vi "2016110576강재원_1번Project.vi"() -> ()   [LabVIEW 2017]
uses:
  <vilib>/DAQmx/read.llb/DAQmx Read (Analog DBL 1Chan 1Samp).vi
  <vilib>/DAQmx/write.llb/DAQmx Write (Digital Bool 1Line 1Point).vi
  <vilib>/DAQmx/write.llb/DAQmx Write (Counter Frequency 1Chan 1Samp).vi
  <vilib>/DAQmx/create/channels.llb/DAQmx Create Channel (DO-Digital Output).vi
  <vilib>/DAQmx/create/channels.llb/DAQmx Create Channel (AI-Voltage-Basic).vi
  <vilib>/DAQmx/create/channels.llb/DAQmx Create Channel (CO-Pulse Generation-Frequency).vi
  <vilib>/DAQmx/configure/timing.llb/DAQmx Timing (Implicit).vi
  <vilib>/DAQmx/miscellaneous.llb/DAQmx Fill In Error Info.vi
panel:
  out "남은 진정제 용량":u8(slide) scale=0.0..100.0
  in  "led4(mad state, 디지털 4번)":tag
  out "위험상태 진입 횟수(5회마다 초기화)":u32(slide) scale=0.0..5.0
  in  "자동 제어 시스템ON/OFF":bool
  out "Danger":bool
  out "Caution":bool
  out "Safe":bool
  out "모터 값(주기점유율)":dbl(knob) scale=0.04..0.1
  in  "모터, pwm(디지털3번)":tag
  in  "led3(GREEN, 디지털2번)":tag
  in  "potentio(아날로그0번)":tag
  out "potemtiometer":dbl(graph)
  in  "led2(RED, 디지털1번)":tag
  in  "시스템 정지":bool
  in  "led1(Yellow, 디지털0번)":tag
  # "STATE"
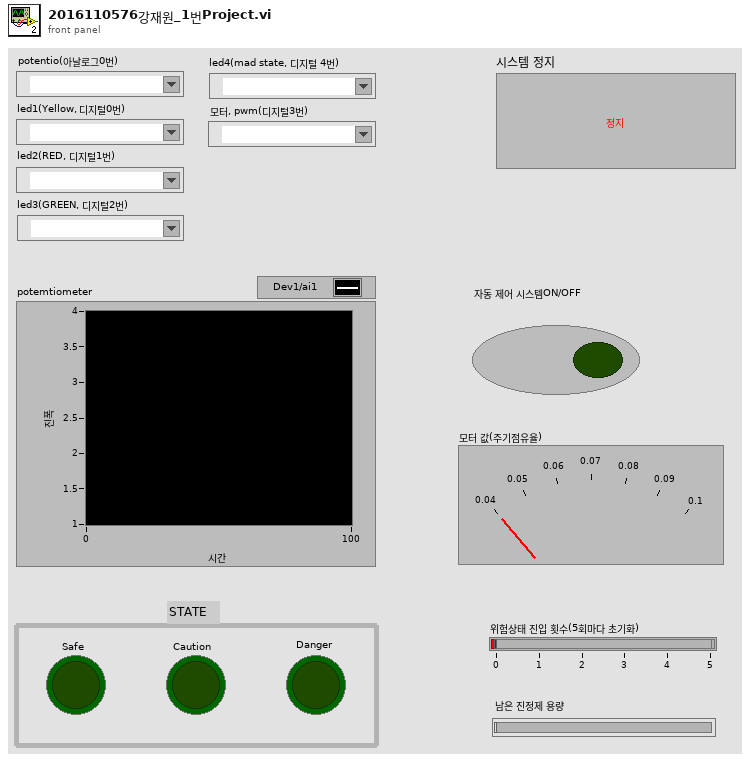
[diagram p1: front panel]
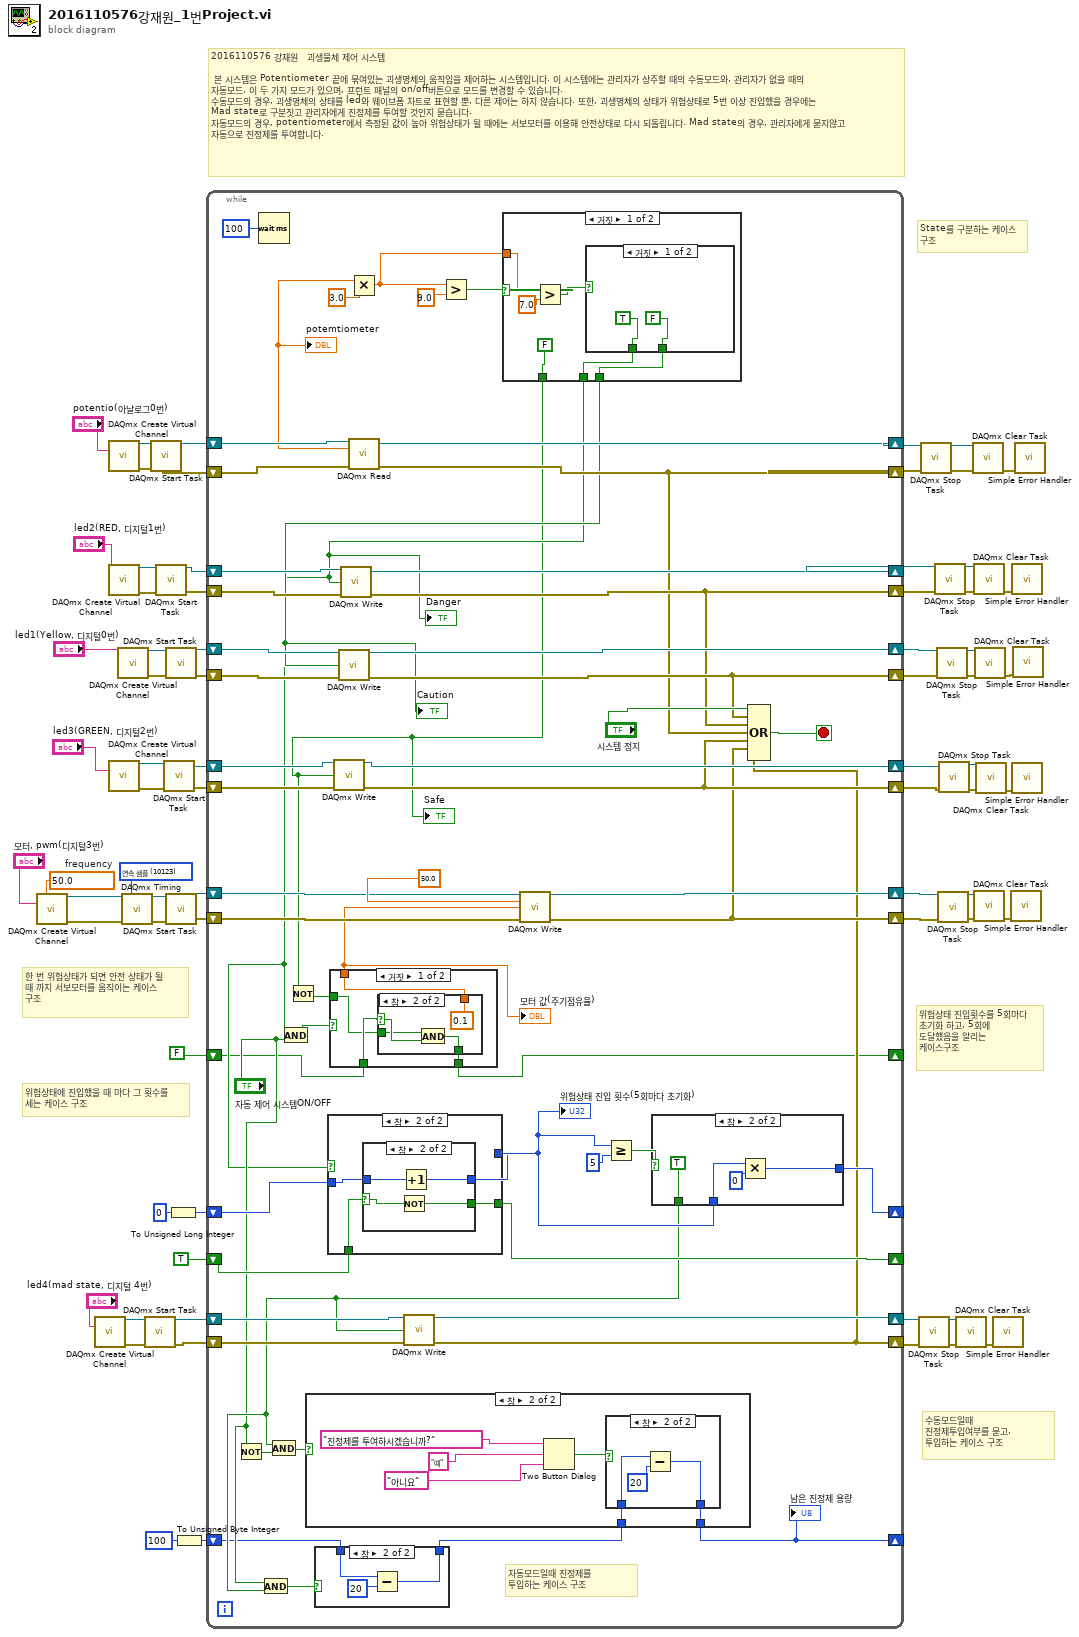
[diagram p0: block diagram]
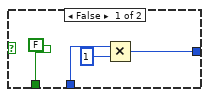
[diagram p5: hidden frame]
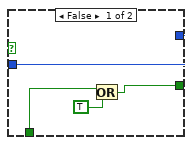
[diagram p6: hidden frame]
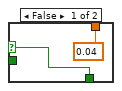
[diagram p8: hidden frame]
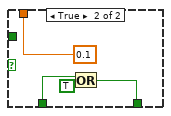
[diagram p9: hidden frame]
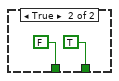
[diagram p10: hidden frame]
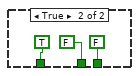
[diagram p11: hidden frame]
diagram:
  w26 = 50.0  # frequency
  w27 = 10123 items=["유한 샘플"=10178, "연속 샘플"=10123, "하드웨어 타이밍에 의한 단일 포인트"=12522] ("sample mode")
  # "수동모드일때 진정제투입여부를 묻고, 투입하는 케이스 구조"
  # "위험상태에 진입했을 때 마다 그 횟수를 세는 케이스 구조"
  # "위험상태 진입횟수를 5회마다 초기화 하고, 5회에 도달했음을 알리는 케이스구조"
  # "한 번 위험상태가 되면 안전 상태가 될 때 까지 서보모터를 움직이는 케이스 구조"
  # "State를 구분하는 케이스 구조"
  # "2016110576 강재원   괴생물체 제어 시스템\n\n 본 시스템은 Potentiometer 끝에 묶여있는 괴생명체의 움직임을 제어하는 시스템입니다. 이 시스템에는 관리자가 상주할 때의 수동모드와, 관리자가 없을 때의 자동모드, 이 두 가지 모드가 있으며, 프런트 패널의 on/off버튼으로 모드를 변경할 수 있습니다.\n수동모드의 경우, 괴생명체의 상태를 led와 웨이브폼 차트로 표현할 뿐, 다른 제어는 하지 않습니다. 또한, 괴생명체의 상태가 위험상태로 5번 이상 진입했을 경우에는 Mad state로 구분짓고 관리자에게 진정제를 투여할 것인지 묻습니다. \n자동모드의 경우, potentiometer에서 측정된 값이 높아 위험상태가 될 때에는 서보모터를 이용해 안전상태로 다시 되돌립니다. Mad state의 경우, 관리자에게 묻지않고 자동으로 진정제를 투여합니다."
  n1 = call-poly <vilib>:"DAQmx Create Virtual Channel.vi"("frequency"=w26, "counter"="모터, pwm(디지털3번)") -> ("task out"=w29:refnum<k21>, "error out"=w30:errorcluster)  [unwired: 12 in]
  n2 = call-poly <vilib>:"DAQmx Create Virtual Channel.vi"("lines"="led4(mad state, 디지털 4번)") -> ("task out"=w10:refnum<k21>, "error out"=w11:errorcluster)  [unwired: 13 in]
  n3 = call-poly <vilib>:"DAQmx Create Virtual Channel.vi"("physical channels"="potentio(아날로그0번)") -> ("task out"=w55:refnum<k21>, "error out"=w54:errorcluster)  [unwired: 13 in]
  n4 = call-poly <vilib>:"DAQmx Create Virtual Channel.vi"("lines"="led2(RED, 디지털1번)") -> ("task out"=w50:refnum<k21>, "error out"=w51:errorcluster)  [unwired: 13 in]
  n5 = call-poly <vilib>:"DAQmx Create Virtual Channel.vi"("lines"="led3(GREEN, 디지털2번)") -> ("task out"=w33:refnum<k21>, "error out"=w34:errorcluster)  [unwired: 13 in]
  n6 = call-poly <vilib>:"DAQmx Create Virtual Channel.vi"("lines"="led1(Yellow, 디지털0번)") -> ("task out"=w65:refnum<k21>, "error out"=w66:errorcluster)  [unwired: 13 in]
  n7 = call-poly <vilib>:"DAQmx Timing.vi"("task/channels in"=w29, "sample mode"=w27, "error in"=w30) -> ("task out"=w28:refnum<k21>, "error out"=w31:errorcluster)  [unwired: 11 in]
  n8 = call <vilib>:"DAQmx Start Task.vi"("task/channels in"=w10, "error in"=w11) -> ("task out"=w8:refnum<k21>, "error out"=w9:errorcluster)  [unwired: 12 in]
  n9 = call <vilib>:"DAQmx Start Task.vi"("task/channels in"=w55, "error in"=w54) -> ("task out"=w56:refnum<k21>, "error out"=w53:errorcluster)  [unwired: 12 in]
  n10 = call <vilib>:"DAQmx Start Task.vi"("task/channels in"=w50, "error in"=w51) -> ("task out"=w43:refnum<k21>, "error out"=w46:errorcluster)  [unwired: 12 in]
  n11 = call <vilib>:"DAQmx Start Task.vi"("task/channels in"=w33, "error in"=w34) -> ("task out"=w37:refnum<k21>, "error out"=w36:errorcluster)  [unwired: 12 in]
  n12 = call <vilib>:"DAQmx Start Task.vi"("task/channels in"=w65, "error in"=w66) -> ("task out"=w63:refnum<k21>, "error out"=w64:errorcluster)  [unwired: 12 in]
  n13 = call <vilib>:"DAQmx Start Task.vi"("task/channels in"=w28, "error in"=w31) -> ("task out"=w18:refnum<k21>, "error out"=w19:errorcluster)  [unwired: 12 in]
  n14 = To Unsigned Long Integer(number=0) -> (unsigned 32bit integer=w16:u32)
  n15 = To Unsigned Byte Integer(number=100) -> (unsigned 8bit integer=w3:u8)
  n16 = while {
    shift-right: [w124] -> w61
    shift-left: w63 -> [w125]
    shift-right: [w114] -> w62
    shift-left: w64 -> [w126]
    shift-right: [w123] -> w57
    shift-left: w56 -> [w122]
    shift-right: [w112] -> w52
    shift-left: w53 -> [w121]
    shift-right: [w119] -> w44
    shift-left: w43 -> [w118]
    shift-right: [w113] -> w45
    shift-left: w46 -> [w120]
    shift-right: [w111] -> w38
    shift-left: w37 -> [w110]
    shift-right: [w108] -> w35
    shift-left: w36 -> [w109]
    shift-right: [w106] -> w21
    shift-left: w18 -> [w104]
    shift-right: [w103] -> w20
    shift-left: w19 -> [w105]
    shift-right: [w90] -> _
    shift-left: w16 -> [w99]
    shift-right: [w97] -> _
    shift-left: TRUE -> [w98]
    shift-right: [w94] -> w7
    shift-left: w8 -> [w95]
    shift-right: [w78] -> w6
    shift-left: w9 -> [w96]
    shift-right: [w87] -> _
    shift-left: w3 -> [w83]
    shift-right: [w75] -> _
    shift-left: FALSE -> [w76]
    stop <- w116 stop-if-true
    # "자동모드일때 진정제를 투입하는 케이스 구조"
    n17 = Not(x="자동 제어 시스템ON/OFF") -> (.not. x?=w88:bool)
    n18 = Wait (ms)(milliseconds to wait=u32 100 ("대기 시간 (ms)")) -> ()  [unwired: 1 out]
    n19 = call-poly <vilib>:"DAQmx Read.vi"("task/channels in"=w122, "error in"=w121) -> ("task out"=w123:refnum<k21>, "data"=w71:dbl, "error out"=w112:errorcluster)  [unwired: 11 in]
    "potemtiometer" <- w71
    n20 = Multiply(x=w71, y=3.0) -> (x*y=w80:dbl)
    n21 = Greater?(x=w80, y=9.0) -> (0:w117:bool)
    n22 = case shown="거짓" w117 {
      tunnel: [w179 FALSE] -> w77
      tunnel: [w180 FALSE] -> w102
      tunnel: w80 -> [w182 _]
      tunnel: [FALSE TRUE] -> w74
      frame False {
        n23 = Greater?(x=w182, y=7.0) -> (0:w181:bool)
        n24 = case shown="거짓" w181 {
          tunnel: [FALSE TRUE] -> w180
          tunnel: [TRUE FALSE] -> w179
          frame False {
          }
          frame True {
          }
        }
      }
      frame True {
      }
    }
    "Safe" <- w74
    "Caution" <- w102
    "Danger" <- w77
    n25 = And(x=w77, y="자동 제어 시스템ON/OFF") -> (x .and. y?=w101:bool)
    n26 = Not(x=w74) -> (.not. x?=w73:bool)
    n27 = case shown="참" w77 {
      tunnel: w99 -> [w153 w157]
      tunnel: [w153 w156] -> w91
      tunnel: w98 -> [w151 w155]
      tunnel: [w150 w154] -> w97
      frame False {
        n28 = Or(x=w151, y=TRUE) -> (x .or. y?=w150:bool)
      }
      frame True {
        n29 = case shown="참" w155 {
          selector: w155 -> [w158 w161]
          tunnel: w157 -> [w159 w163]
          tunnel: [w159 w162] -> w156
          tunnel: [w158 w160] -> w154
          frame False {
          }
          frame True {
            n30 = Not(x=w161) -> (.not. x?=w160:bool)
            n31 = Increment(x=w163) -> (x+1=w162:u32)
          }
        }
      }
    }
    "위험상태 진입 횟수(5회마다 초기화)" <- w91
    n32 = case shown="거짓" w101 {
      tunnel: [w166 0.1] -> w72
      tunnel: w76 -> [w167 w175]
      tunnel: [w165 w174] -> w75
      tunnel: w73 -> [w164 _]
      frame False {
        n33 = case shown="참" w167 {
          selector: w167 -> [w168 w171]
          tunnel: [0.04 0.1] -> w166
          tunnel: [w168 w172] -> w165
          tunnel: w164 -> [_ w170]
          frame False {
          }
          frame True {
            n34 = And(x=w170, y=w171) -> (x .and. y?=w172:bool)
          }
        }
      }
      frame True {
        n35 = Or(x=w175, y=TRUE) -> (x .or. y?=w174:bool)
      }
    }
    "모터 값(주기점유율)" <- w72
    n36 = call-poly <vilib>:"DAQmx Write.vi"("task/channels in"=w110, "data"=w74, "error in"=w109) -> ("task out"=w111:refnum<k21>, "error out"=w108:errorcluster)  [unwired: 10 in, 1 out]
    n37 = call-poly <vilib>:"DAQmx Write.vi"("task/channels in"=w125, "data"=w102, "error in"=w126) -> ("task out"=w124:refnum<k21>, "error out"=w114:errorcluster)  [unwired: 10 in, 1 out]
    n38 = call-poly <vilib>:"DAQmx Write.vi"("task/channels in"=w118, "data"=w77, "error in"=w120) -> ("task out"=w119:refnum<k21>, "error out"=w113:errorcluster)  [unwired: 10 in, 1 out]
    n39 = call-poly <vilib>:"DAQmx Write.vi"("task/channels in"=w104, "frequency"=50.0, "duty cycle"=w72, "error in"=w105) -> ("task out"=w106:refnum<k21>, "error out"=w103:errorcluster)  [unwired: 9 in, 1 out]
    n40 = Greater Or Equal?(x=w91, y=u32 5) -> (x >= y?=w92:bool)
    n41 = case shown="참" w92 {
      tunnel: [FALSE TRUE] -> w86
      tunnel: w91 -> [w144 w148]
      tunnel: [w142 w146] -> w90
      frame False {
        n42 = Multiply(x=w144, y=u32 1) -> (x*y=w142:u32)
      }
      frame True {
        n43 = Multiply(x=w148, y=u32 0) -> (x*y=w146:u32)
      }
    }
    n44 = And(x="자동 제어 시스템ON/OFF", y=w86) -> (x .and. y?=w85:bool)
    n45 = And(x=w86, y=w88) -> (x .and. y?=w89:bool)
    n46 = case shown="참" w85 {
      tunnel: w83 -> [w127 w130]
      tunnel: [w127 w128] -> w82
      frame False {
      }
      frame True {
        n47 = Subtract(x=w130, y=u8 20) -> (x-y=w128:u8)
      }
    }
    n48 = case shown="참" w89 {
      tunnel: w82 -> [w131 w133]
      tunnel: [w131 w132] -> w87
      frame False {
      }
      frame True {
        n49 = Two Button Dialog(message="진정제를 투여하시겠습니까?" ("메시지"), 1:"아니요" ("거짓 버튼 이름(\"취소\")"), 2:"예" ("참 버튼 이름(\"확인\")")) -> (T button?=w134:bool)
        n50 = case shown="참" w134 {
          tunnel: w133 -> [w138 w141]
          tunnel: [w138 w139] -> w132
          frame False {
          }
          frame True {
            n51 = Subtract(x=w141, y=u8 20) -> (x-y=w139:u8)
          }
        }
      }
    }
    "남은 진정제 용량" <- w87
    n52 = call-poly <vilib>:"DAQmx Write.vi"("task/channels in"=w95, "data"=w86, "error in"=w96) -> ("task out"=w94:refnum<k21>, "error out"=w78:errorcluster)  [unwired: 10 in, 1 out]
    n53 = Compound Arithmetic op=OR("시스템 정지", w114, w113, w112, w108, w103, w78) -> (w116:bool)
  }
  n54 = call <vilib>:"DAQmx Stop Task.vi"("task/channels in"=w7, "error in"=w6) -> ("task out"=w12:refnum<k21>, "error out"=w13:errorcluster)  [unwired: 12 in]
  n55 = call <vilib>:"DAQmx Stop Task.vi"("task/channels in"=w57, "error in"=w52) -> ("task out"=w58:refnum<k21>, "error out"=w59:errorcluster)  [unwired: 12 in]
  n56 = call <vilib>:"DAQmx Stop Task.vi"("task/channels in"=w44, "error in"=w45) -> ("task out"=w47:refnum<k21>, "error out"=w49:errorcluster)  [unwired: 12 in]
  n57 = call <vilib>:"DAQmx Stop Task.vi"("task/channels in"=w61, "error in"=w62) -> ("task out"=w68:refnum<k21>, "error out"=w70:errorcluster)  [unwired: 12 in]
  n58 = call <vilib>:"DAQmx Stop Task.vi"("task/channels in"=w21, "error in"=w20) -> ("task out"=w22:refnum<k21>, "error out"=w23:errorcluster)  [unwired: 12 in]
  n59 = call <vilib>:"DAQmx Stop Task.vi"("task/channels in"=w38, "error in"=w35) -> ("task out"=w39:refnum<k21>, "error out"=w40:errorcluster)  [unwired: 12 in]
  n60 = call <vilib>:"DAQmx Clear Task.vi"("task in"=w12, "error in"=w13) -> ("error out"=w14:errorcluster)  [unwired: 13 in]
  n61 = call <vilib>:"DAQmx Clear Task.vi"("task in"=w58, "error in"=w59) -> ("error out"=w60:errorcluster)  [unwired: 13 in]
  n62 = call <vilib>:"DAQmx Clear Task.vi"("task in"=w47, "error in"=w49) -> ("error out"=w48:errorcluster)  [unwired: 13 in]
  n63 = call <vilib>:"DAQmx Clear Task.vi"("task in"=w22, "error in"=w23) -> ("error out"=w24:errorcluster)  [unwired: 13 in]
  n64 = call <vilib>:"DAQmx Clear Task.vi"("task in"=w68, "error in"=w70) -> ("error out"=w69:errorcluster)  [unwired: 13 in]
  n65 = call <vilib>:"DAQmx Clear Task.vi"("task in"=w39, "error in"=w40) -> ("error out"=w41:errorcluster)  [unwired: 13 in]
  n66 = call <vilib>:"Simple Error Handler.vi"("error in (no error)"=w14) -> ()  [unwired: 4 in, 5 out]
  n67 = call <vilib>:"Simple Error Handler.vi"("error in (no error)"=w24) -> ()  [unwired: 4 in, 5 out]
  n68 = call <vilib>:"Simple Error Handler.vi"("error in (no error)"=w48) -> ()  [unwired: 4 in, 5 out]
  n69 = call <vilib>:"Simple Error Handler.vi"("error in (no error)"=w41) -> ()  [unwired: 4 in, 5 out]
  n70 = call <vilib>:"Simple Error Handler.vi"("error in (no error)"=w69) -> ()  [unwired: 4 in, 5 out]
  n71 = call <vilib>:"Simple Error Handler.vi"("error in (no error)"=w60) -> ()  [unwired: 4 in, 5 out]
